vi "gen angle array.vi"(8 "Invert":bool, 9 "angular step":dbl=-45.0, 10 "angle start":dbl=-45.0, 11 "array size":i32=811) -> (3 "output array":dbl[](array[numeric]))   [LabVIEW 2017]
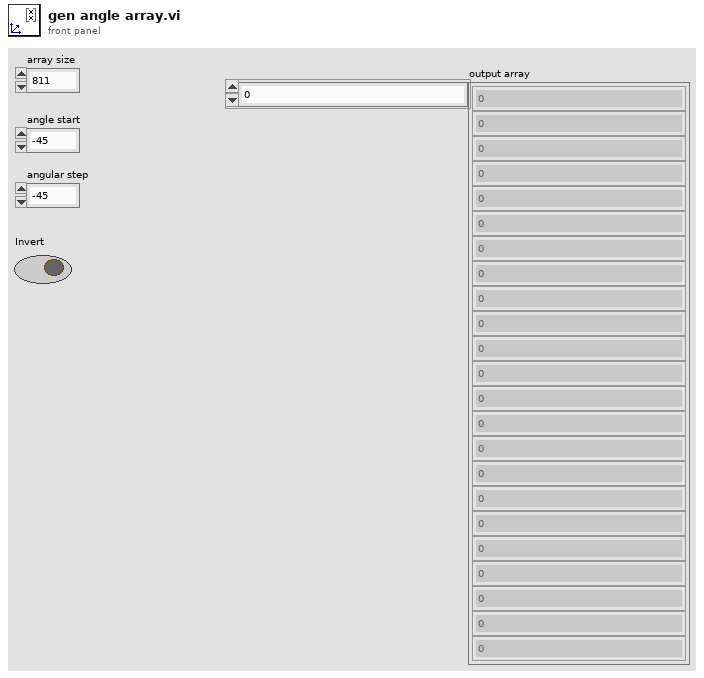
[diagram p1: front panel]
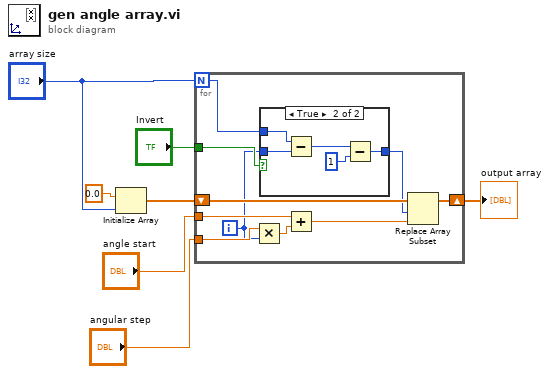
[diagram p0: block diagram]
diagram:
  n1 = Initialize Array(0.0 ("element"), "array size") -> (w6:dbl[])
  n2 = for {
    N: "array size" -> [w8]
    shift-right: [w16] -> w5
    shift-left: w6 -> [w17]
    tunnel: "angular step" -> [w15]
    tunnel: "angle start" -> [w13]
    tunnel: "Invert" -> [w11]
    i -> [w10]
    n3 = Multiply(x=w15, y=w10) -> (x*y=w14:dbl)
    n4 = case shown="True" w11 {
      tunnel: [w18 w20] -> w9
      tunnel: w10 -> [w18 w22]
      tunnel: w8 -> [_ w23]
      frame False {
      }
      frame True {
        n5 = Subtract(x=w23, y=w22) -> (x-y=w21:i32)
        n6 = Subtract(x=w21, y=1) -> (x-y=w20:i32)
      }
    }
    n7 = Add(x=w13, y=w14) -> (x+y=w12:dbl)
    n8 = Replace Array Subset(array=w17, new element=w12, index=w9) -> (w16:dbl[])
  }
  "output array" <- w5
